vi "Move AxisX DistY.vi"() -> ()   [LabVIEW 2015]
uses:
  <userlib>/Newport ESP301/Newport ESP301.lvlib
panel:
  in  "Axis":i32
  in  "Movement":dbl
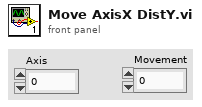
[diagram p1: front panel]
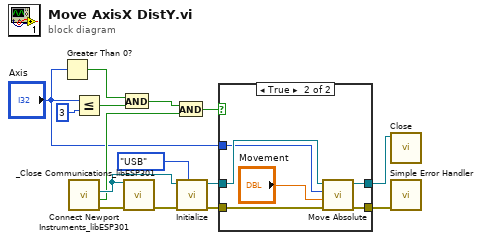
[diagram p0: block diagram]
diagram:
  n1 = Greater Than 0?(x="Axis") -> (x > 0?=w5:bool)
  n2 = call <userlib>:"Connect Newport Instruments_libESP301.vi"() -> ("error (duplicate)"=w13:errorcluster, "Connected"=w4:bool, "VISA resource name (duplicate)"=w12:refnum<visa-resource-name>)  [unwired: 7 in, 2 out]
  n3 = Less Or Equal?(x="Axis", y=3) -> (x <= y?=w6:bool)
  n4 = And(x=w5, y=w6) -> (x .and. y?=w3:bool)
  n5 = call <userlib>:"_Close Communications_libESP301.vi"("Instrument Channel"=w12, "error in (no error)"=w13) -> ("error out"=w15:errorcluster)  [unwired: 13 in]
  n6 = And(x=w3, y=w4) -> (x .and. y?=w2:bool)
  n7 = call <userlib>:"Initialize.vi"("VISA resource name"=w12, "error in (no error)"=w15, "Serial Link (USB)"=enum16{"RS232", "USB"}."USB" ("Serial Link (RS232)")) -> ("VISA resource name out"=w11:refnum<visa-resource-name>, "error out"=w10:errorcluster)  [unwired: 6 in]
  n8 = case shown="True" w2 {
    tunnel: w11 -> [w17 w22]
    tunnel: w10 -> [w16 w23]
    tunnel: [w17 w18] -> w9
    tunnel: [w16 w19] -> w8
    tunnel: "Axis" -> [_ w20]
    frame False {
    }
    frame True {
      n9 = call <userlib>:"Move Absolute.vi"("error in (no error)"=w23, "Position (0 units)"="Movement", "Axis (1)"=w20, "VISA resource name"=w22) -> ("error out"=w19:errorcluster, "VISA resource name out"=w18:refnum<visa-resource-name>)  [unwired: 2 in]
    }
  }
  n10 = call <userlib>:"Close.vi"("VISA resource name"=w9) -> ()  [unwired: 10 in, 1 out]
  n11 = call <vilib>:"Simple Error Handler.vi"("error in (no error)"=w8) -> ()  [unwired: 1 in, 8 out]
